vi "FP place the boat.vi"(2 "Y pos":i32=100, 3 "X pos":i32=100, 4 "Boat image\nPixels (U32)":u32[][](array[numeric]), 5 "Pool image\nPixels (U32)":u32[][](array[numeric])) -> (1 "Pool image\nPixels (U32) out":u32[][](array[numeric]))   [LabVIEW 2014]
doc: "This vi will place the boat image in the pool image based upon the X and Y position. It will create a color image array. The position is not valid if the boat is within a solid."
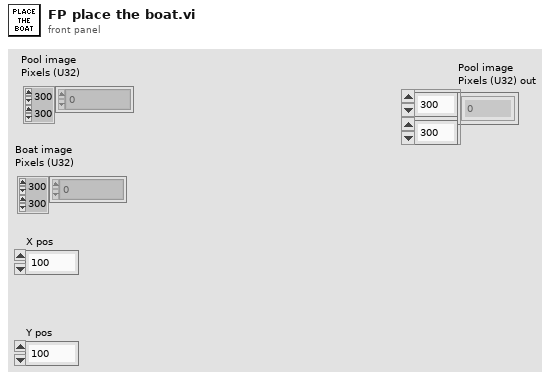
[diagram p1: front panel]
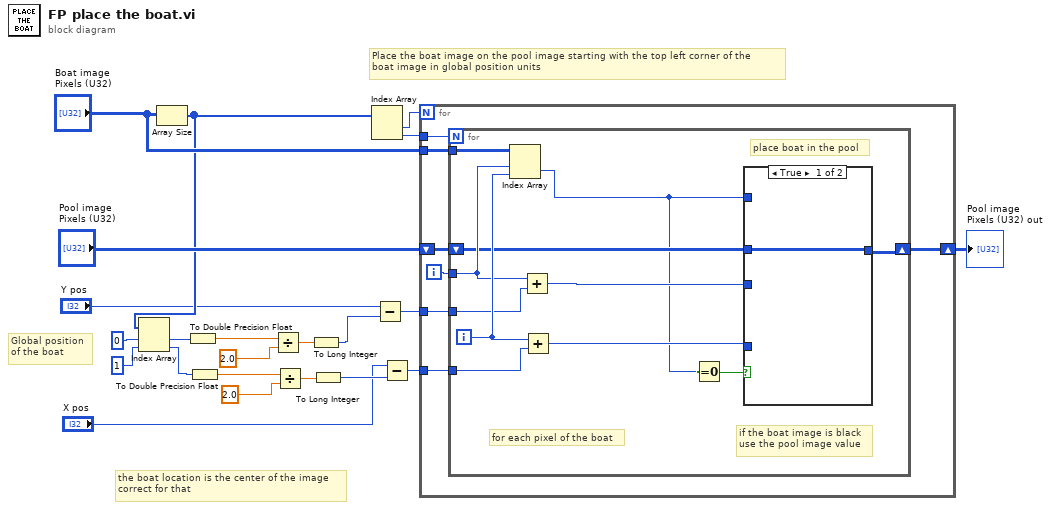
[diagram p0: block diagram]
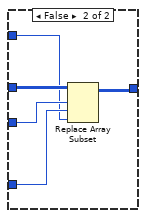
[diagram p2: hidden frame]
diagram:
  # "Place the boat image on the pool image starting with the top left corner of the\nboat image in global position units"
  # "Global position\nof the boat"
  # "the boat location is the center of the image\ncorrect for that"
  n1 = Array Size(array="Boat image\nPixels (U32)") -> (size(s)=w7:i32[])
  n2 = Index Array(array=w7, index #1=0 ("index"), index #2=1 ("index")) -> (element #1=w14:i32, element #2=w10:i32)
  n3 = To Double Precision Float(number=w14) -> (double precision float=w13:dbl)
  n4 = To Double Precision Float(number=w10) -> (double precision float=w11:dbl)
  n5 = Divide(x=w13, y=2.0) -> (x/y=w9:dbl)
  n6 = Divide(x=w11, y=2.0) -> (x/y=w8:dbl)
  n7 = To Long Integer(number=w9) -> (32bit integer=w5:i32)
  n8 = To Long Integer(number=w8) -> (32bit integer=w2:i32)
  n9 = Index Array(array=w7) -> (element #1=w22:i32, element #2=w21:i32)  [unwired: 2 in]
  n10 = Subtract(x="Y pos", y=w5) -> (x-y=w4:i32)
  n11 = Subtract(x="X pos", y=w2) -> (x-y=w3:i32)
  n12 = for {
    N: w22 -> [_]
    tunnel: w21 -> [w28]
    tunnel: "Boat image\nPixels (U32)" -> [w27]
    shift-right: [w25] -> w18
    shift-left: "Pool image\nPixels (U32)" -> [w26]
    tunnel: w4 -> [w24]
    tunnel: w3 -> [w23]
    i -> [w29]
    n13 = for {
      N: w28 -> [_]
      tunnel: w29 -> [w39]
      tunnel: w27 -> [w32]
      shift-right: [w38] -> w25
      shift-left: w26 -> [w36]
      tunnel: w24 -> [w35]
      tunnel: w23 -> [w34]
      i -> [w40]
      # "for each pixel of the boat"
      # "if the boat image is black\nuse the pool image value"
      # "place boat in the pool"
      n14 = Index Array(array=w32, index (row)=w39, index (col)=w40) -> (element=w30:u32)
      n15 = Add(x=w39, y=w35) -> (x+y=w33:i32)
      n16 = Add(x=w40, y=w34) -> (x+y=w37:i32)
      n17 = Equal To 0?(x=w30) -> (x = 0?=w31:bool)
      n18 = case shown="True" w31 {
        tunnel: [w41 w46] -> w38
        tunnel: w33 -> [_ w45]
        tunnel: w37 -> [_ w44]
        tunnel: w36 -> [w41 w43]
        tunnel: w30 -> [_ w42]
        frame True {
        }
        frame False {
          n19 = Replace Array Subset(array=w43, new element=w42, index (row)=w45, index (col)=w44) -> (w46:u32[][])
        }
      }
    }
  }
  "Pool image\nPixels (U32) out" <- w18
